vi "Store New Connection.vi"(7 "Connection Reference":refnum<data-value>, 8 "error in (no error)":errorcluster, 9 "Active Connection ID":string, 10 "Connection Manager Queue":refnum<class "Message Enqueuer.lvclass">, 11 "PersistantConnectionHandler in":refnum<class "PersistantConnectionHandler.lvclass">) -> (0 "error out":errorcluster, 3 "PersistantConnectionHandler out":refnum<class "PersistantConnectionHandler.lvclass">)   [LabVIEW 2019, in "PersitantConnectionHandler.lvlib" / "PersistantConnectionHandler.lvclass"]
uses:
  <vilib>/gpm_packages/@cs/Network-interface/Source/PersistantConnectionHandler/PersistantConnectionHandler/PersistantConnectionHandler.lvclass
  <vilib>/ActorFramework/Message Enqueuer/Message Enqueuer.lvclass
  <vilib>/gpm_packages/@cs/Network-interface/Source/Connection Reference/Connection Reference/Connection Reference.lvclass
  <vilib>/gpm_packages/@cs/Network-interface/Source/PersistantConnectionHandler/PersistantConnectionHandler/PersistantConnectionHandler.lvclass/PersistantConnectionHandler.ctl
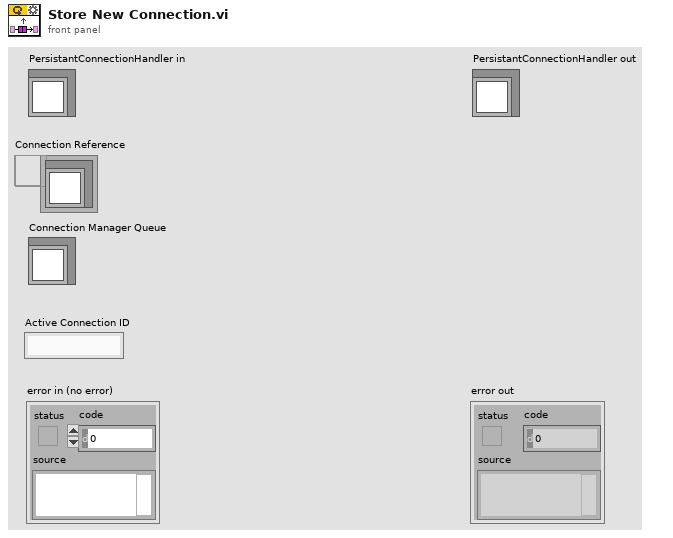
[diagram p1: front panel]
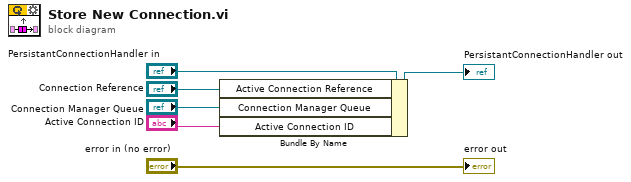
[diagram p0: block diagram]
diagram:
  n1 = Bundle By Name(cluster="PersistantConnectionHandler in", "Active Connection Reference"="Connection Reference", "Connection Manager Queue"="Connection Manager Queue", "Active Connection ID"="Active Connection ID") -> (→"PersistantConnectionHandler out":refnum<class "PersistantConnectionHandler.lvclass">)
  "error out" <- "error in (no error)"
